vi "Populate Tree From Folder.vi"(10 "Folder Path":path) -> (3 "Tree":string(tree))   [LabVIEW 2025]
panel:
  out "File Items":T1(array[cluster])
  out "Folder Items":T1(array[cluster])
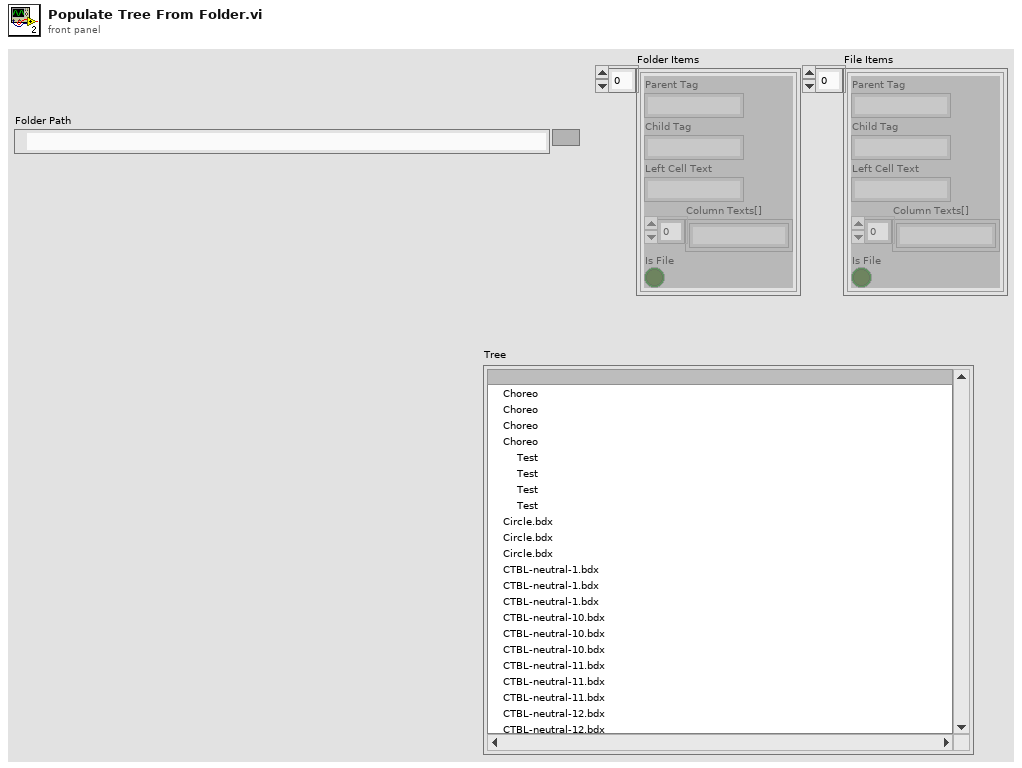
[diagram p1: front panel]
types:
  T1 = cluster{"Parent Tag":string, "Child Tag":string, "Left Cell Text":string, "Column Texts[]":string[], "Is File":bool}[]
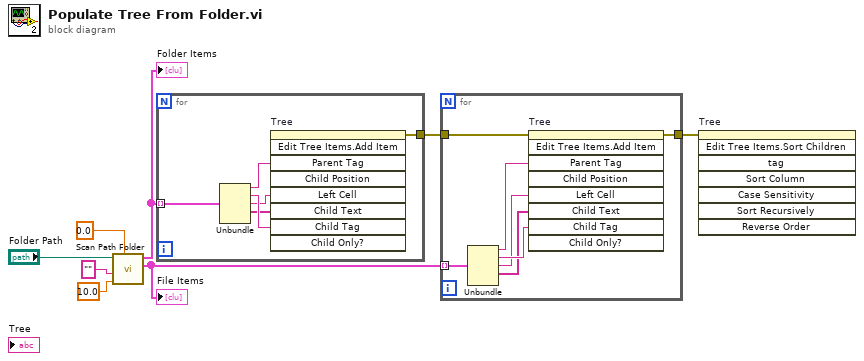
[diagram p0: block diagram]
diagram:
  n1 = call "Scan Path Folder.vi"("Current Depth"=0.0, "Max Depth"=10.0, "Parent Tag"="", "Path"="Folder Path") -> ("File Items"=w3:T1, "Folder Items"=w4:T1)  [unwired: 6 in]
  "Folder Items" <- w4
  "File Items" <- w3
  n2 = for {
    tunnel: w4 -> [w14] mode=indexing
    tunnel: [w9] -> w2
    n3 = Unbundle(w14) -> ("Parent Tag"=w13:string, "Child Tag"=w12:string, "Left Cell Text"=w11:string, "Column Texts[]"=w10:string[])  [unwired: 1 out]
    n4 = invoke on="Tree" class="Tree (strict)" method="Edit Tree Items.Add Item"("Parent Tag"=w13, "Left Cell"=w11, "Child Text"=w10, "Child Tag"=w12) -> (error out=w9:errorcluster)  [unwired: 5 in, 8 out]
  }
  n5 = for {
    tunnel: w3 -> [w21] mode=indexing
    tunnel: w2 -> [w16]
    tunnel: [w15] -> w1
    n6 = Unbundle(w21) -> ("Parent Tag"=w20:string, "Child Tag"=w19:string, "Left Cell Text"=w18:string, "Column Texts[]"=w17:string[])  [unwired: 1 out]
    n7 = invoke on="Tree" class="Tree (strict)" method="Edit Tree Items.Add Item"(error in=w16, "Parent Tag"=w20, "Left Cell"=w18, "Child Text"=w17, "Child Tag"=w19) -> (error out=w15:errorcluster)  [unwired: 4 in, 8 out]
  }
  n8 = invoke on="Tree" class="Tree (strict)" method="Edit Tree Items.Sort Children"(error in=w1) -> ()  [unwired: 7 in, 8 out]
